vi "Get DC Motors.vi"(8 "error in (no error)":errorcluster, 11 "NI_Robotics_Starter Kit Host in":refnum<class "NI_Robotics_Starter Kit Host.lvclass">) -> (0 "error out":errorcluster, 1 "DC motor 1 (right)":refnum<class "DC Motor Controller.lvclass">, 2 "DC motor 0 (left)":refnum<class "DC Motor Controller.lvclass">, 3 "NI_Robotics_Starter Kit Host out":refnum<class "NI_Robotics_Starter Kit Host.lvclass">)   [LabVIEW 2017, in "NI_Robotics_Starter Kit Host.lvclass"]
uses:
  <vilib>/robotics/Starter Kit/Host Interface/NI_Robotics_Starter Kit Host.lvclass
  <instrlib>/DC Motor Controller/HAIOL/DC Motor Controller.lvclass
  <vilib>/robotics/Starter Kit/Host Interface/NI_Robotics_Starter Kit Host.lvclass/NI_Robotics_Starter Kit Host.ctl
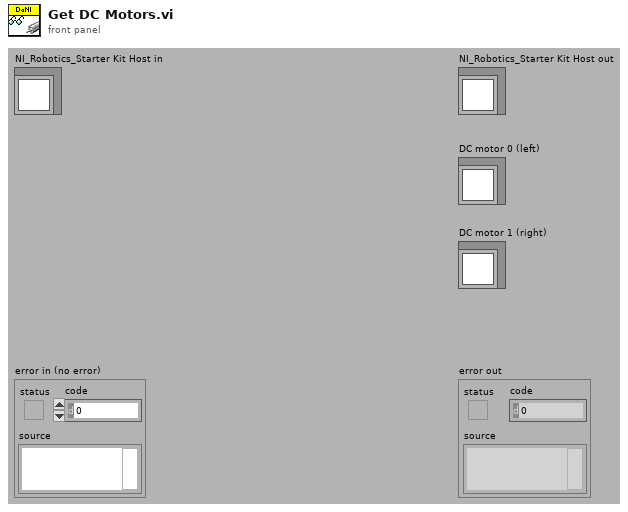
[diagram p1: front panel]
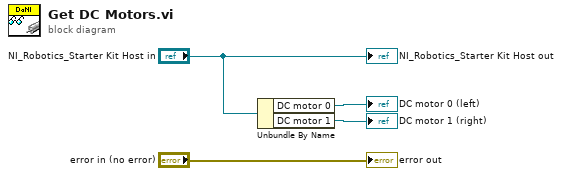
[diagram p0: block diagram]
diagram:
  n1 = Unbundle By Name("NI_Robotics_Starter Kit Host in") -> ("DC motor 0"=→"DC motor 0 (left)":refnum<class "DC Motor Controller.lvclass">, "DC motor 1"=→"DC motor 1 (right)":refnum<class "DC Motor Controller.lvclass">)
  "error out" <- "error in (no error)"
  "NI_Robotics_Starter Kit Host out" <- "NI_Robotics_Starter Kit Host in"
